vi "XYZStage-Request move.vi"(7 "Current State":T1, 9 "Pos ctrl window queue":refnum<queue>, 10 "Previous State":T1, 11 "variant":variant) -> ()   [LabVIEW 2020]
uses:
  User Interface/Windows/Position control window/Typedefs/Pos Ctrl queue data cluster.ctl
  User Interface/Windows/Position control window/Typedefs/Pos Ctrl States.ctl
  User Interface/Windows/Position control window/Globals/Pos ctrl window globals.vi
panel:
  out "x+1":dbl
  out "Button name":string
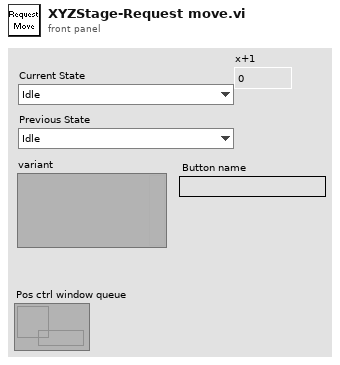
[diagram p1: front panel]
types:
  T1 = typedef "Pos Ctrl States.ctl" = enum16{"Idle", "Count-down", "Request single step (ack.)", "Request single step (no ack.)", "Request continuous movement", "Request movement stop"}
  T2 = typedef "Movement mode.ctl" = enum16{"Move the frame", "Move the feature"}
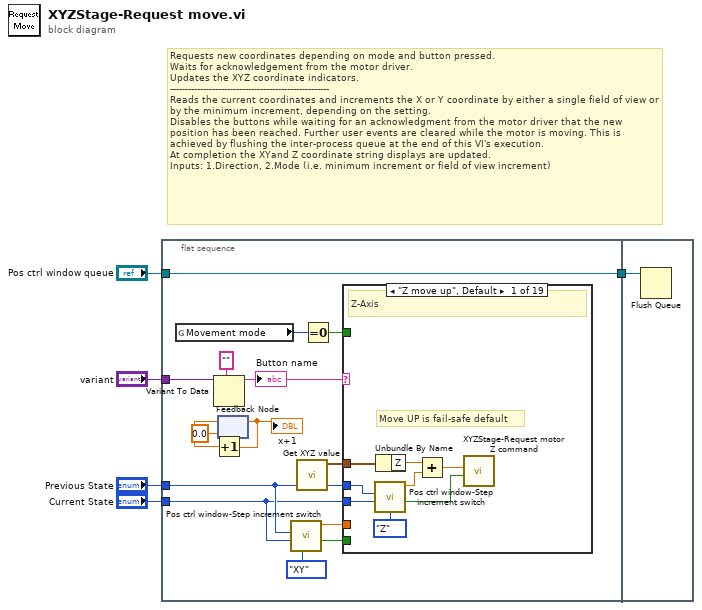
[diagram p0: block diagram]
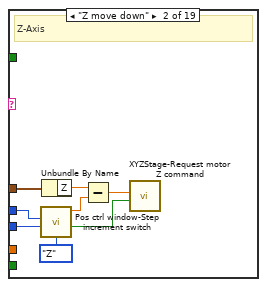
[diagram p2: hidden frame]
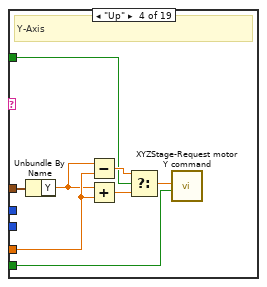
[diagram p4: hidden frame]
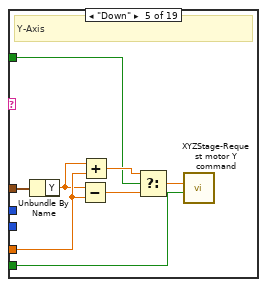
[diagram p5: hidden frame]
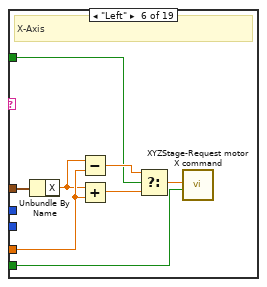
[diagram p6: hidden frame]
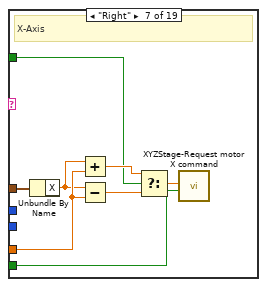
[diagram p7: hidden frame]
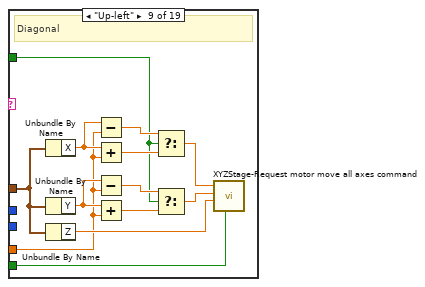
[diagram p9: hidden frame]
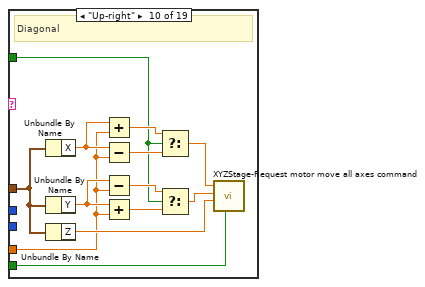
[diagram p10: hidden frame]
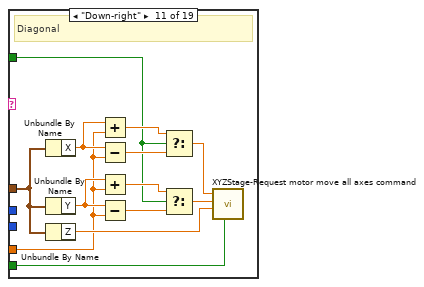
[diagram p11: hidden frame]
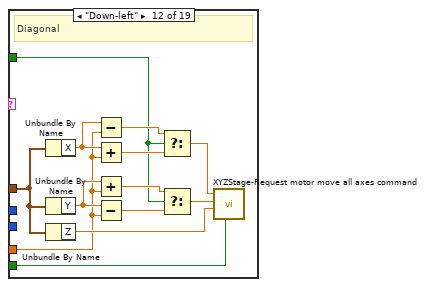
[diagram p12: hidden frame]
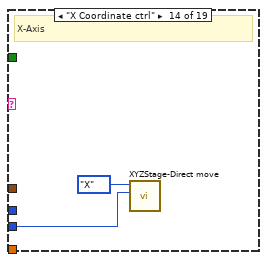
[diagram p14: hidden frame]
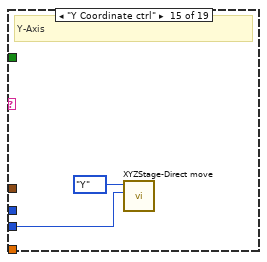
[diagram p15: hidden frame]
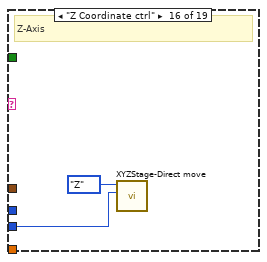
[diagram p16: hidden frame]
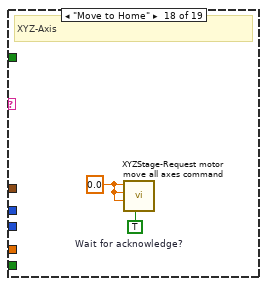
[diagram p18: hidden frame]
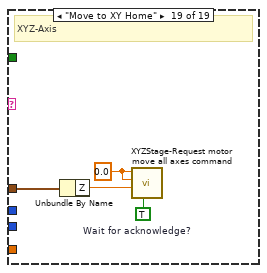
[diagram p19: hidden frame]
diagram:
  # "Requests new coordinates depending on mode and button pressed.\nWaits for acknowledgement from the motor driver.\nUpdates the XYZ coordinate indicators.\n-----------------------------------------------------\nReads the current coordinates and increments the X or Y coordinate by either a single field of view or by the minimum increment, depending on the setting.\nDisables the buttons while waiting for an acknowledgment from the motor driver that the new position has been reached. Further user events are cleared while the motor is moving. This is achieved by flushing the inter-process queue at the end of this VI's execution.\nAt completion the XYand Z coordinate string displays are updated.\nInputs: 1.Direction, 2.Mode (i.e. minimum increment or field of view increment)"
  n1 = flat-sequence {
    tunnel: [w18] -> w5
    tunnel: "Pos ctrl window queue" -> [w18]
    tunnel: "Previous State" -> [w14]
    tunnel: "variant" -> [w16]
    tunnel: "Current State" -> [w11]
    tunnel: w5 -> [w133]
    frame #0 {
      n2 = global read "Pos ctrl window globals.vi" "Movement mode"() -> (w7:T2)
      n3 = Variant To Data(type="" ("Label.Text"), Variant=w16) -> (data=w19:string)  [unwired: 1 in, 1 out]
      "Button name" <- w19
      n4 = feedback #1(0.0) -> (w9:dbl)
      n5 = Increment(x=w9) -> (x+1=w10:dbl)
      "x+1" <- w10
      n6 = feedback-in #1(w10) -> ()
      n7 = call "Pos ctrl window-Step increment switch.vi"("Mode"=enum16{"XY", "Z"}."XY", "State"=w11, "Previous State"=w14) -> ("Wait for acknowledge?"=w13:bool, "Increment (um)"=w17:sgl)  [unwired: 7 in]
      n8 = call "Get XYZ value.vi"() -> ("Stage XYZ Position"=w12:cluster{"X":sgl, "Y":sgl, "Z":sgl})  [unwired: 11 in]
      n9 = Equal To 0?(x=w7) -> (x = 0?=w6:bool)
      n10 = case shown="\"Z move up\", Default" w19 {
        tunnel: w12 -> [w28 w36 _ w44 w52 w60 w68 _ w81 w94 w107 w120 _ _ _ _ _ _ w130]
        tunnel: w17 -> [_ _ _ w40 w51 w56 w64 _ w71 w84 w98 w109 _ _ _ _ _ _ _]
        tunnel: w14 -> [w24 w32 _ _ _ _ _ _ _ _ _ _ _ _ _ _ _ _ _]
        tunnel: w11 -> [w23 w31 _ _ _ _ _ _ _ _ _ _ _ w121 w123 w125 _ _ _]
        tunnel: w13 -> [_ _ _ w43 w46 w59 w67 _ w79 w92 w105 w118 _ _ _ _ _ _ _]
        tunnel: w6 -> [_ _ _ w37 w45 w53 w61 _ w69 w82 w95 w108 _ _ _ _ _ _ _]
        frame "Z move up", Default {
          # "Move UP is fail-safe default"
          # "Z-Axis"
          n11 = call "Pos ctrl window-Step increment switch.vi"("Mode"=enum16{"XY", "Z"}."Z", "State"=w23, "Previous State"=w24) -> ("Wait for acknowledge?"=w21:bool, "Increment (um)"=w22:sgl)  [unwired: 7 in]
          n12 = Unbundle By Name(w28) -> ("Z"=w27:sgl)
          n13 = Add(x=w27, y=w22) -> (x+y=w26:sgl)
          n14 = call "XYZStage-Request motor Z command.vi"("Wait for acknowledge?"=w21, "Motor Z"=w26) -> ()  [unwired: 7 in, 3 out]
        }
        frame "Z move down" {
          # "Z-Axis"
          n15 = call "Pos ctrl window-Step increment switch.vi"("Mode"=enum16{"XY", "Z"}."Z", "State"=w31, "Previous State"=w32) -> ("Wait for acknowledge?"=w29:bool, "Increment (um)"=w30:sgl)  [unwired: 7 in]
          n16 = Unbundle By Name(w36) -> ("Z"=w35:sgl)
          n17 = Subtract(x=w35, y=w30) -> (x-y=w34:sgl)
          n18 = call "XYZStage-Request motor Z command.vi"("Wait for acknowledge?"=w29, "Motor Z"=w34) -> ()  [unwired: 7 in, 3 out]
        }
        frame "[XY axis movement cases below]" {
        }
        frame "Up" {
          # "Y-Axis"
          n19 = Unbundle By Name(w44) -> ("Y"=w39:sgl)
          n20 = Subtract(x=w39, y=w40) -> (x-y=w38:sgl)
          n21 = Add(x=w39, y=w40) -> (x+y=w42:sgl)
          n22 = Select(t=w38, s=w37, f=w42) -> (s? t:f=w41:sgl)
          n23 = call "XYZStage-Request motor Y command.vi"("Wait for acknowledge?"=w43, "Motor Y"=w41) -> ()  [unwired: 8 in, 2 out]
        }
        frame "Down" {
          # "Y-Axis"
          n24 = Unbundle By Name(w52) -> ("Y"=w50:sgl)
          n25 = Subtract(x=w50, y=w51) -> (x-y=w48:sgl)
          n26 = Add(x=w50, y=w51) -> (x+y=w49:sgl)
          n27 = Select(t=w49, s=w45, f=w48) -> (s? t:f=w47:sgl)
          n28 = call "XYZStage-Request motor Y command.vi"("Wait for acknowledge?"=w46, "Motor Y"=w47) -> ()  [unwired: 8 in, 2 out]
        }
        frame "Left" {
          # "X-Axis"
          n29 = Unbundle By Name(w60) -> ("X"=w55:sgl)
          n30 = Subtract(x=w55, y=w56) -> (x-y=w54:sgl)
          n31 = Add(x=w55, y=w56) -> (x+y=w57:sgl)
          n32 = Select(t=w54, s=w53, f=w57) -> (s? t:f=w58:sgl)
          n33 = call "XYZStage-Request motor X command.vi"("Wait for acknowledge?"=w59, "Motor X"=w58) -> ()  [unwired: 8 in, 2 out]
        }
        frame "Right" {
          # "X-Axis"
          n34 = Unbundle By Name(w68) -> ("X"=w63:sgl)
          n35 = Add(x=w63, y=w64) -> (x+y=w62:sgl)
          n36 = Subtract(x=w63, y=w64) -> (x-y=w66:sgl)
          n37 = Select(t=w62, s=w61, f=w66) -> (s? t:f=w65:sgl)
          n38 = call "XYZStage-Request motor X command.vi"("Wait for acknowledge?"=w67, "Motor X"=w65) -> ()  [unwired: 8 in, 2 out]
        }
        frame "[Diagonal movement cases below]" {
        }
        frame "Up-left" {
          # "Diagonal"
          n39 = Unbundle By Name(w81) -> ("X"=w74:sgl)
          n40 = Unbundle By Name(w81) -> ("Y"=w72:sgl)
          n41 = Unbundle By Name(w81) -> ("Z"=w80:sgl)
          n42 = Subtract(x=w74, y=w71) -> (x-y=w73:sgl)
          n43 = Add(x=w74, y=w71) -> (x+y=w78:sgl)
          n44 = Subtract(x=w72, y=w71) -> (x-y=w70:sgl)
          n45 = Add(x=w72, y=w71) -> (x+y=w77:sgl)
          n46 = Select(t=w73, s=w69, f=w78) -> (s? t:f=w76:sgl)
          n47 = Select(t=w70, s=w69, f=w77) -> (s? t:f=w75:sgl)
          n48 = call "XYZStage-Request motor move all axes command.vi"("Wait for acknowledge?"=w79, "Motor Z"=w80, "Motor Y"=w75, "Motor X"=w76) -> ()  [unwired: 6 in, 2 out]
        }
        frame "Up-right" {
          # "Diagonal"
          n49 = Unbundle By Name(w94) -> ("X"=w87:sgl)
          n50 = Unbundle By Name(w94) -> ("Y"=w85:sgl)
          n51 = Unbundle By Name(w94) -> ("Z"=w93:sgl)
          n52 = Add(x=w87, y=w84) -> (x+y=w86:sgl)
          n53 = Subtract(x=w87, y=w84) -> (x-y=w88:sgl)
          n54 = Subtract(x=w85, y=w84) -> (x-y=w83:sgl)
          n55 = Add(x=w85, y=w84) -> (x+y=w89:sgl)
          n56 = Select(t=w86, s=w82, f=w88) -> (s? t:f=w91:sgl)
          n57 = Select(t=w83, s=w82, f=w89) -> (s? t:f=w90:sgl)
          n58 = call "XYZStage-Request motor move all axes command.vi"("Wait for acknowledge?"=w92, "Motor Z"=w93, "Motor Y"=w90, "Motor X"=w91) -> ()  [unwired: 6 in, 2 out]
        }
        frame "Down-right" {
          # "Diagonal"
          n59 = Unbundle By Name(w107) -> ("X"=w100:sgl)
          n60 = Unbundle By Name(w107) -> ("Y"=w99:sgl)
          n61 = Unbundle By Name(w107) -> ("Z"=w106:sgl)
          n62 = Add(x=w100, y=w98) -> (x+y=w96:sgl)
          n63 = Subtract(x=w100, y=w98) -> (x-y=w101:sgl)
          n64 = Add(x=w99, y=w98) -> (x+y=w97:sgl)
          n65 = Subtract(x=w99, y=w98) -> (x-y=w102:sgl)
          n66 = Select(t=w96, s=w95, f=w101) -> (s? t:f=w104:sgl)
          n67 = Select(t=w97, s=w95, f=w102) -> (s? t:f=w103:sgl)
          n68 = call "XYZStage-Request motor move all axes command.vi"("Wait for acknowledge?"=w105, "Motor Z"=w106, "Motor Y"=w103, "Motor X"=w104) -> ()  [unwired: 6 in, 2 out]
        }
        frame "Down-left" {
          # "Diagonal"
          n69 = Unbundle By Name(w120) -> ("X"=w111:sgl)
          n70 = Unbundle By Name(w120) -> ("Y"=w110:sgl)
          n71 = Unbundle By Name(w120) -> ("Z"=w119:sgl)
          n72 = Subtract(x=w111, y=w109) -> (x-y=w112:sgl)
          n73 = Add(x=w111, y=w109) -> (x+y=w115:sgl)
          n74 = Add(x=w110, y=w109) -> (x+y=w113:sgl)
          n75 = Subtract(x=w110, y=w109) -> (x-y=w114:sgl)
          n76 = Select(t=w112, s=w108, f=w115) -> (s? t:f=w117:sgl)
          n77 = Select(t=w113, s=w108, f=w114) -> (s? t:f=w116:sgl)
          n78 = call "XYZStage-Request motor move all axes command.vi"("Wait for acknowledge?"=w118, "Motor Z"=w119, "Motor Y"=w116, "Motor X"=w117) -> ()  [unwired: 6 in, 2 out]
        }
        frame "[Direct numerical entry buttons]" {
        }
        frame "X Coordinate ctrl" {
          # "X-Axis"
          n79 = call "XYZStage-Direct move.vi"("Current State"=w121, "Coordinate to set"=enum16{"X", "Y", "Z"}."X") -> ()  [unwired: 8 in, 2 out]
        }
        frame "Y Coordinate ctrl" {
          # "Y-Axis"
          n80 = call "XYZStage-Direct move.vi"("Current State"=w123, "Coordinate to set"=enum16{"X", "Y", "Z"}."Y") -> ()  [unwired: 8 in, 2 out]
        }
        frame "Z Coordinate ctrl" {
          # "Z-Axis"
          n81 = call "XYZStage-Direct move.vi"("Current State"=w125, "Coordinate to set"=enum16{"X", "Y", "Z"}."Z") -> ()  [unwired: 8 in, 2 out]
        }
        frame "[Menu commands below]" {
        }
        frame "Move to Home" {
          w128 = TRUE  # Wait for acknowledge?
          w127 = sgl 0.0 ("Motor X")
          # "XYZ-Axis"
          n82 = call "XYZStage-Request motor move all axes command.vi"("Wait for acknowledge?"=w128, "Motor Z"=w127, "Motor Y"=w127, "Motor X"=w127) -> ()  [unwired: 6 in, 2 out]
        }
        frame "Move to XY Home" {
          w132 = TRUE  # Wait for acknowledge?
          w131 = sgl 0.0 ("Motor X")
          # "XYZ-Axis"
          n83 = Unbundle By Name(w130) -> ("Z"=w129:sgl)
          n84 = call "XYZStage-Request motor move all axes command.vi"("Wait for acknowledge?"=w132, "Motor Z"=w129, "Motor Y"=w131, "Motor X"=w131) -> ()  [unwired: 6 in, 2 out]
        }
      }
    }
    frame #1 {
      n85 = Flush Queue(queue=w133) -> ()  [unwired: 1 in, 3 out]
    }
  }
